vi "AlliGator Load Single HDF5 Gate Image v 0.2b.vi"(6 "Action":T1, 8 "error in (no error)":errorcluster, 10 "File Info":variant, 11 "Gate Index":i32) -> (0 "error out":errorcluster, 1 "Data 2":sgl[][](array[numeric]), 3 "Data 1":sgl[][](array[numeric]))   [LabVIEW 2021, in "AlliGator HDF5.lvlib"]
doc: "Loads single gate image from HDF5 FLI dataset file (v0.2)."
uses:
  AlliGator HDF5.lvlib
  AlliGator FLI Image Stack Action.ctl
  AlliGator HDF5 FLI File Loading Information v0.2.ctl
  <vilib>/addons/h5labview2/base/lib_path.vi
  <vilib>/addons/h5labview2/base/H5Equery.vi
  <vilib>/Utility/error.llb/Error Cluster From Error Code.vi
  <vilib>/addons/h5labview2/base/hid_t.ctl
  <vilib>/addons/h5labview2/dataset/H5Dread.llb/H5Dread.xnode
  <vilib>/ErrorRing/Error Ring.xnode
  <vilib>/addons/h5labview2/file/H5F.lvlib
panel:
  # "see the AlliGator License on the block diagram (Ctrl+E or Window:Show Block Diagram)"
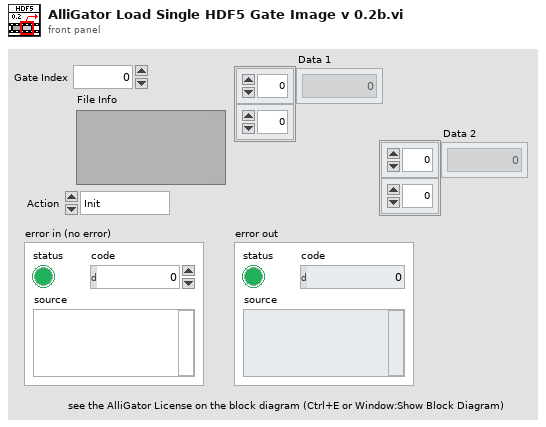
[diagram p1: front panel]
types:
  T1 = typedef "AlliGator HDF5.lvlib/AlliGator FLI Image Stack Action.ctl" = enum16{"Init", "Get Image", "Close"}
  T2 = typedef "AlliGator HDF5.lvlib/AlliGator HDF5 FLI File Loading Information v0.2.ctl" = cluster{"HDF5 File Path":path}
  T3 = typedef "hid_t.ctl" = i64
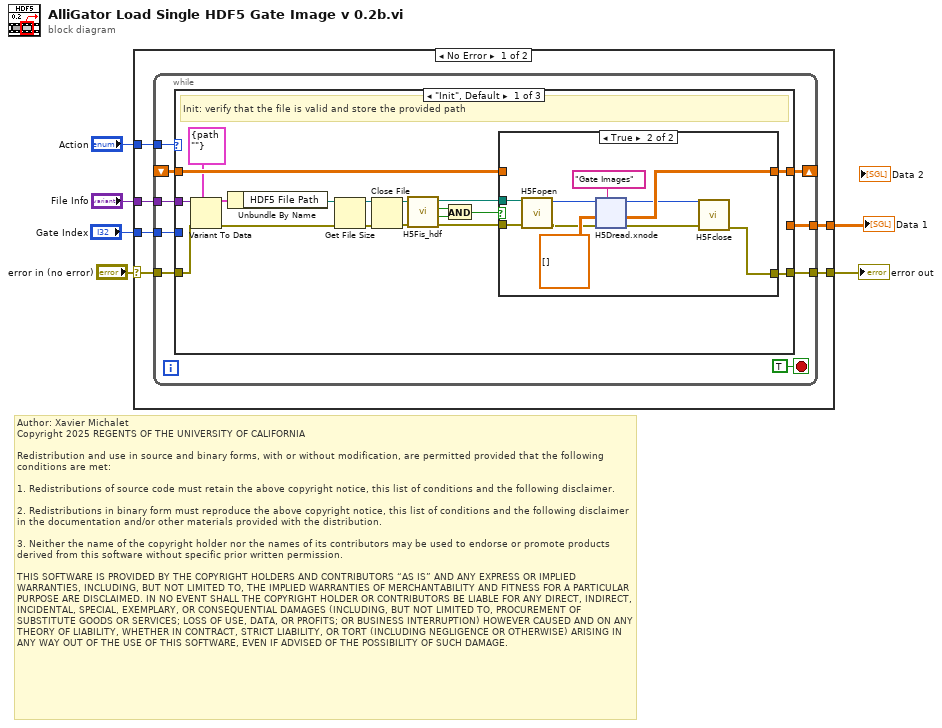
[diagram p0: block diagram]
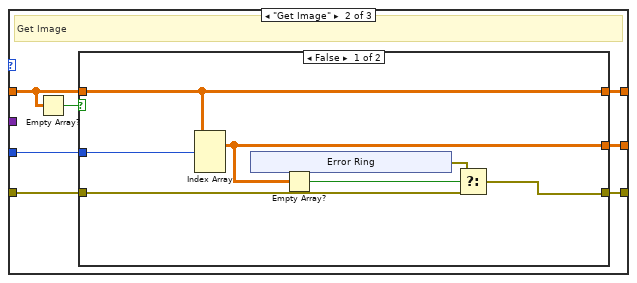
[diagram p3: hidden frame]
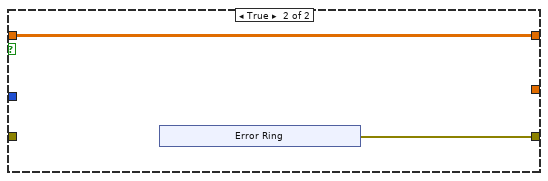
[diagram p4: hidden frame]
diagram:
  # "Author: Xavier Michalet\nCopyright 2025 REGENTS OF THE UNIVERSITY OF CALIFORNIA\n\nRedistribution and use in source and binary forms, with or without modification, are permitted provided that the following conditions are met:\n\n1. Redistributions of source code must retain the above copyright notice, this list of conditions and the following disclaimer.\n\n2. Redistributions in binary form must reproduce the above copyright notice, this list of conditions and the following disclaimer in the documentation and/or other materials provided with the distribution.\n\n3. Neither the name of the copyright holder nor the names of its contributors may be used to endorse or promote products derived from this software without specific prior written permission.\n\nTHIS SOFTWARE IS PROVIDED BY THE COPYRIGHT HOLDERS AND CONTRIBUTORS “AS IS” AND ANY EXPRESS OR IMPLIED WARRANTIES, INCLUDING, BUT NOT LIMITED TO, THE IMPLIED WARRANTIES OF MERCHANTABILITY AND FITNESS FOR A PARTICULAR PURPOSE ARE DISCLAIMED. IN NO EVENT SHALL THE COPYRIGHT HOLDER OR CONTRIBUTORS BE LIABLE FOR ANY DIRECT, INDIRECT, INCIDENTAL, SPECIAL, EXEMPLARY, OR CONSEQUENTIAL DAMAGES (INCLUDING, BUT NOT LIMITED TO, PROCUREMENT OF SUBSTITUTE GOODS OR SERVICES; LOSS OF USE, DATA, OR PROFITS; OR BUSINESS INTERRUPTION) HOWEVER CAUSED AND ON ANY THEORY OF LIABILITY, WHETHER IN CONTRACT, STRICT LIABILITY, OR TORT (INCLUDING NEGLIGENCE OR OTHERWISE) ARISING IN ANY WAY OUT OF THE USE OF THIS SOFTWARE, EVEN IF ADVISED OF THE POSSIBILITY OF SUCH DAMAGE."
  n1 = case shown="No Error" "error in (no error)" {
    selector: "error in (no error)" -> [w11 w92]
    tunnel: [w10 w92] -> w5
    tunnel: "Action" -> [w12 _]
    tunnel: "File Info" -> [w9 _]
    tunnel: "Gate Index" -> [w8 _]
    tunnel: [w7 _] -> w1
    frame No Error {
      n2 = while {
        tunnel: w12 -> [w20]
        tunnel: w11 -> [w19]
        tunnel: [w18] -> w10
        tunnel: w9 -> [w17]
        shift-right: [w16] -> _
        shift-left: _ -> [w15]
        tunnel: w8 -> [w14]
        tunnel: [w13] -> w7
        stop <- TRUE stop-if-true
        n3 = case shown="\"Init\", Default" w20 {
          tunnel: w19 -> [w25 w69 w91]
          tunnel: [w28 w72 w91] -> w18
          tunnel: w17 -> [w27 _ _]
          tunnel: [w30 w73 _] -> w16
          tunnel: w15 -> [w29 w71 _]
          tunnel: w14 -> [_ w68 _]
          tunnel: [_ w67 _] -> w13
          frame "Init", Default {
            # "Init: verify that the file is valid and store the provided path"
            n4 = Variant To Data(error in=w25, type=T2 {"HDF5 File Path"=path ""} ("HDF5 FLI File Loading Information"), Variant=w27) -> (data=w23:T2, error out=w26:errorcluster)
            n5 = Unbundle By Name(w23) -> ("HDF5 File Path"=w22:path)
            n6 = Get File Size(file=w22, error in=w26) -> (refnum out=w36:refnum<file>, 0:w37:errorcluster)  [unwired: 1 out]
            n7 = Close File(refnum=w36, error in=w37) -> (path=w35:path, error out=w34:errorcluster)
            n8 = call <vilib>:"H5Fis_hdf.vi"("error in (no error)"=w34, "path in"=w35) -> ("error out"=w32:errorcluster, "valid?"=w38:bool, "exists?"=w39:bool, "path out"=w31:path)  [unwired: 6 in]
            n9 = And(x=w39, y=w38) -> (x .and. y?=w33:bool)
            n10 = case shown="True" w33 {
              tunnel: w32 -> [w40 w48]
              tunnel: w31 -> [_ w49]
              tunnel: [w41 w45] -> w30
              tunnel: w29 -> [w41 _]
              tunnel: [w40 w42] -> w28
              frame False {
              }
              frame True {
                n11 = call <vilib>:"H5Fopen.vi"("error in (no error)"=w48, "path"=w49) -> ("error out"=w46:errorcluster, "ref out"=w47:T3)  [unwired: 8 in]
                n12 = xnode "H5Dread.xnode"("dataset name (this)"="Gate Images" ("dataset name"), "error in (no error)"=w46, "default"=sgl[][][] [] ("Data"), "ref in"=w47) -> ("error out"=w43:errorcluster, "data"=w45:sgl[][][], "ref out"=w44:T3)  [unwired: 2 in, 1 out]
                n13 = call <vilib>:"H5Fclose.vi"("error in (no error)"=w43, "ref"=w44) -> ("error out"=w42:errorcluster)  [unwired: 9 in]
              }
            }
          }
          frame "Get Image" {
            # "Get Image"
            n14 = Empty Array?(array=w71) -> (empty?=w70:bool)
            n15 = case shown="False" w70 {
              tunnel: [w79 w86] -> w73
              tunnel: w71 -> [w79 w86]
              tunnel: [w75 w85] -> w72
              tunnel: w69 -> [w76 _]
              tunnel: w68 -> [w80 _]
              tunnel: [w78 _] -> w67
              frame False {
                n16 = Index Array(array=w79, index (dim 0)=w80) -> (element=w78:sgl[][])  [unwired: 2 in]
                n17 = xnode "Error Ring"() -> ("error out"=w74:errorcluster)
                n18 = Empty Array?(array=w78) -> (empty?=w77:bool)
                n19 = Select(t=w74, s=w77, f=w76) -> (s? t:f=w75:errorcluster)
              }
              frame True {
                n20 = xnode "Error Ring"() -> ("error out"=w85:errorcluster)
              }
            }
          }
          frame "Close" {
            # "Close File"
          }
        }
      }
    }
    frame Error {
    }
  }
  "Data 1" <- w1
  "error out" <- w5
